vi "__Alicat SD_ManualSetFlows.vi"(1 "SET FLOW":dbl[](array[numeric])=[0.0, 0.0] format="%.2f", 6 "error in (no error)":errorcluster, 9 "COMMS":T1={"Alicats"="ASRL6::INSTR", "Alic"=FALSE, "eValve"="ASRL6::INSTR", "eval"=FALSE, "Eurotherm"="ASRL6::INSTR", "euro"=FALSE, "Cell GAS"="ASRL6::INSTR", "cgas"=FALSE, "Cell H2S"="ASRL6::INSTR", "ch2s"=FALSE}) -> (0 "error out":errorcluster, 3 "Cancelled?":bool)   [LabVIEW 2017]
doc: "Use this template to create a dialog box. This template polls the state of the buttons on the front panel and does not use events. Use the Dialog Using Events template (not available in Base package) to create a dialog box with event handling."
uses:
  __s_TablaAlicats.ctl
  REACTOR_COMUNICACIONES.ctl
  REACTOR_GLOBALES.vi
panel:
  in  "Canal4":bool
  in  "Canal3":bool
  out "ID":string[](array[string])
  out "CONECTADO":bool[](array[boolean])
  in  "Canal2":bool
  in  "Canal1":bool
  out "aDispositivos":T2=[["A", "NO", "aM0000013", "Air", "100", "ln/mn", "0.1", "0.11"], ["B", "NO", "aM0000014", "Air", "100", "ln/mn", "0.2", "0.22"], ["C", "NO", "aM0000015", "Air", "100", "ln/mn", "0.3", "0.33"], ["D", "NO", "aM0000016", "Air", "500", "ln/mn", "0.4", "0.44"]] caption="Alicats"
  out "RANGOS":dbl[](array[numeric]) format="%.1g"
  in  "Cancel":bool
  in  "OK":bool
  # "Nota: \nAl hacer CLICK en el botón aparecerá\nla ventana para establecer el nuevo setpoint"
  # "Flujos Alicats"
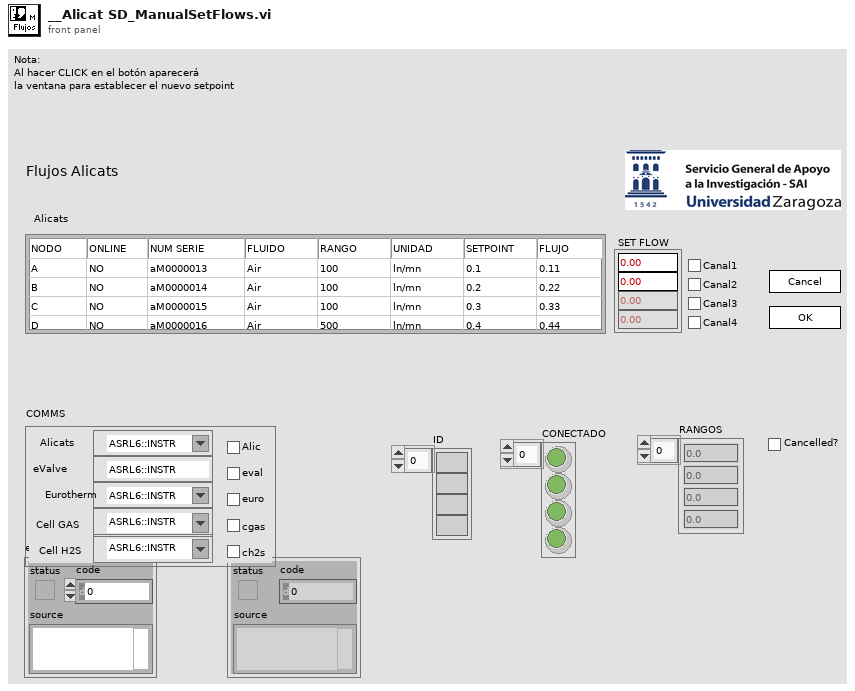
[diagram p1: front panel]
types:
  T1 = typedef "REACTOR_COMUNICACIONES.ctl" = cluster{"Alicats":refnum<visa-resource-name>, "Alic":bool, "eValve":refnum<visa-resource-name>, "eval":bool, "Eurotherm":refnum<visa-resource-name>, "euro":bool, "Cell GAS":refnum<visa-resource-name>, "cgas":bool, "Cell H2S":refnum<visa-resource-name>, "ch2s":bool}
  T2 = typedef "__s_TablaAlicats.ctl" = string[][]
  T3 = typedef "__s_SPali4.ctl" = cluster{"Ch1":dbl, "Ch2":dbl, "Ch3":dbl, "Ch4":dbl}
  T4 = cluster{"SETPOINT 2[0]":dbl, "SETPOINT 2[1]":dbl, "SETPOINT 2[2]":dbl, "SETPOINT 2[3]":dbl}
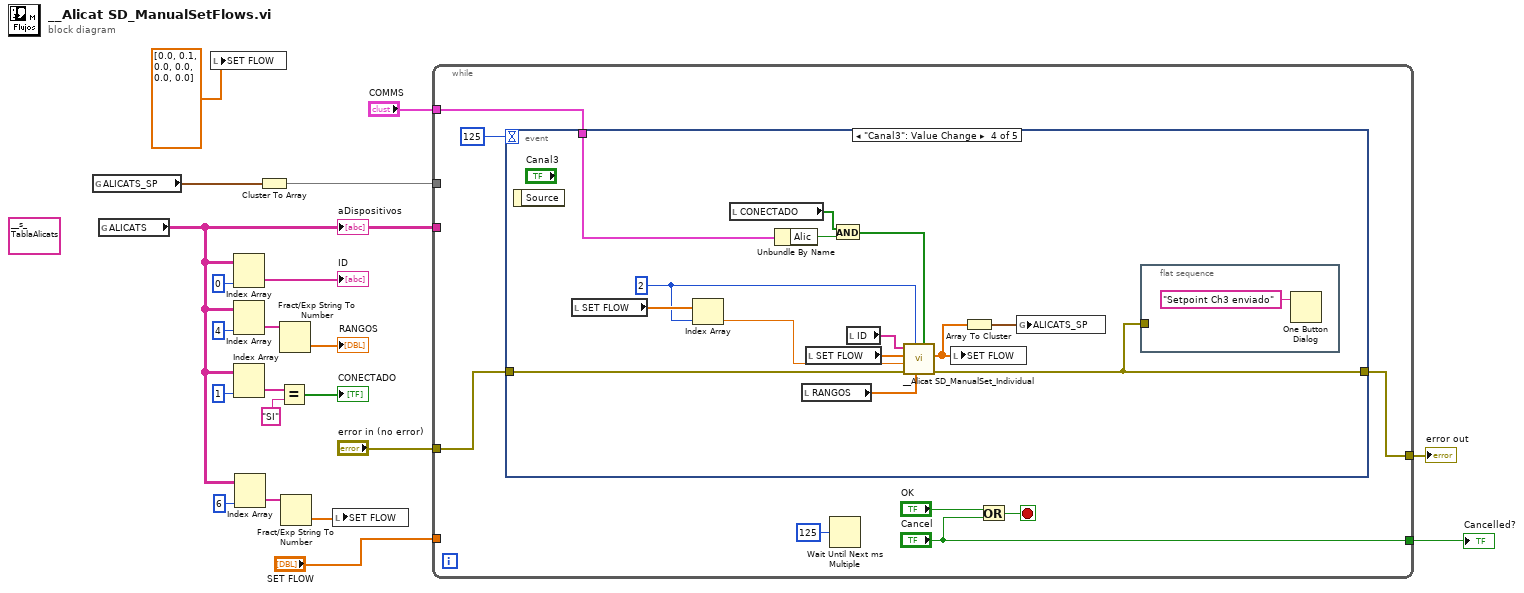
[diagram p0: block diagram]
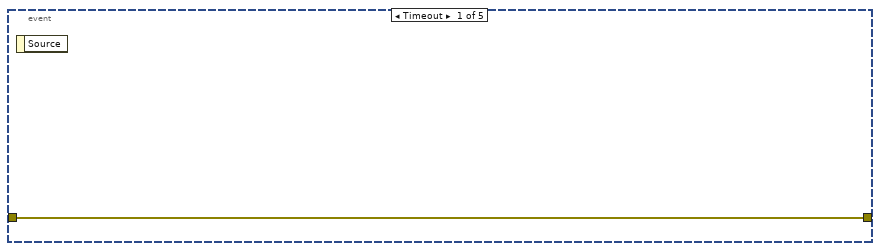
[diagram p2: hidden frame]
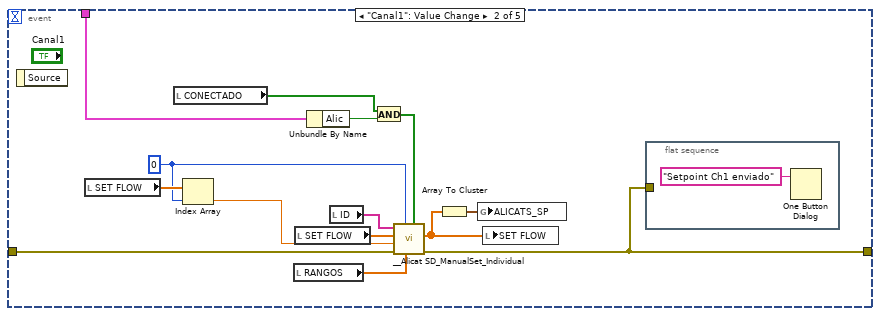
[diagram p3: hidden frame]
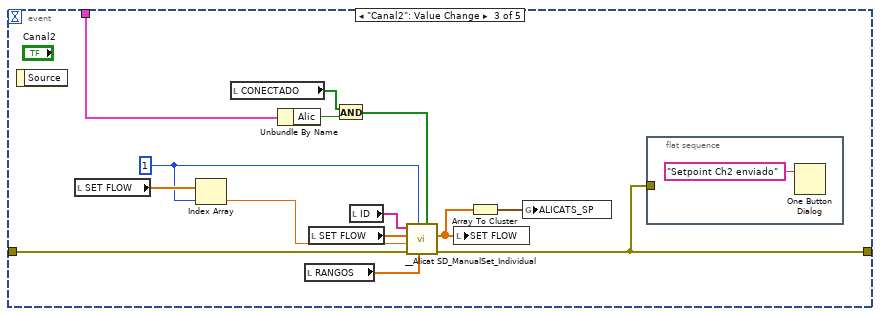
[diagram p4: hidden frame]
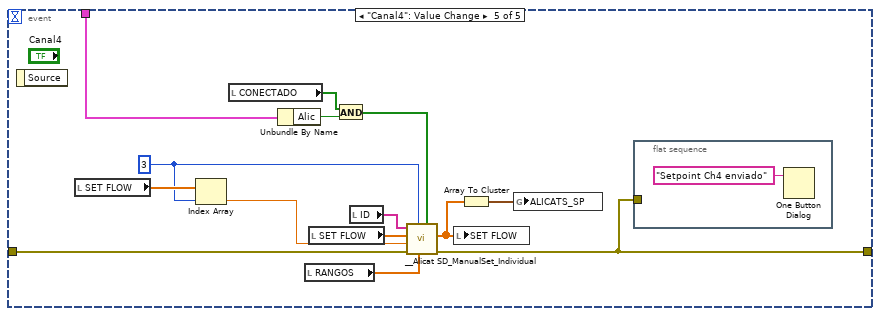
[diagram p5: hidden frame]
diagram:
  (unwired) T2 [["3", "NO", "aM0000013", "Air", "1", "ln/mn", "0.1", "0.11"], ["4", "NO", "aM0000014", "Air", "1", "ln/mn", "0.2", "0.22"], ["5", "NO", "aM0000015", "Air", "1", "ln/mn", "0.3", "0.33"], ["6", "NO", "aM0000016", "Air", "1", "ln/mn", "0.4", "0.44"]] ("Dispositivos 2")
  n1 = global read "REACTOR_GLOBALES.vi" "ALICATS_SP"() -> (w9:T3)
  n2 = global read "REACTOR_GLOBALES.vi" "ALICATS"() -> (w3:T2)
  "aDispositivos" <- w3
  n3 = local write "SET FLOW"(dbl[] [0.0, 0.1, 0.0, 0.0, 0.0, 0.0] ("SET FLOW")) -> ()
  n4 = Index Array(array=w3, index (col)=0 ("disabled index (col)")) -> (element=→"ID":string[])  [unwired: 1 in]
  n5 = Index Array(array=w3, index (col)=4 ("disabled index (col)")) -> (element=w19:string[])  [unwired: 1 in]
  n6 = Index Array(array=w3, index (col)=1 ("disabled index (col)")) -> (element=w12:string[])  [unwired: 1 in]
  n7 = Index Array(array=w3, index (col)=6 ("disabled index (col)")) -> (element=w5:string[])  [unwired: 1 in]
  n8 = Cluster To Array(cluster=w9) -> (array=w7:dbl[])
  n9 = Equal?(x=w12, y="SI") -> (x = y?=→"CONECTADO":bool[])
  n10 = Fract/Exp String To Number(string=w19) -> (number=→"RANGOS":dbl[])  [unwired: 3 in, 1 out]
  n11 = Fract/Exp String To Number(string=w5) -> (number=w1:dbl[])  [unwired: 3 in, 1 out]
  n12 = local write "SET FLOW"(w1) -> ()
  n13 = while {
    tunnel: ["Cancel"] -> w21
    tunnel: "error in (no error)" -> [w24]
    tunnel: [w23] -> w16
    tunnel: w3 -> [_]
    tunnel: "COMMS" -> [w22]
    tunnel: w7 -> [_]
    tunnel: "SET FLOW" -> [_]
    stop <- w28 stop-if-true
    n14 = event shown="[3] \"Canal3\": Value Change" {
      selector: _ -> [_ _ _ _ _]
      dyn-events: _ -> [_ _ _ _ _]
      timeout: 125 -> [_ _ _ _ _]
      tunnel: w24 -> [w30 w32 w47 w63 w78]
      tunnel: [w30 w31 w46 w61 w76] -> w23
      tunnel: w22 -> [_ w34 w49 w64 w79]
      event Timeout {
        n15 = event-data() -> ()  [unwired: 1 in, 1 out]
      }
      event "Canal1": Value Change {
        w40 = 0 ("Address (0.7)")
        n16 = event-data() -> ()  [unwired: 1 in, 1 out]
        n17 = local read "SET FLOW"() -> (w41:dbl[])
        n18 = local read "CONECTADO"() -> (w38:bool[])
        n19 = Index Array(array=w41, index=w40) -> (element=w33:dbl)
        n20 = local read "RANGOS"() -> (w44:dbl[])
        n21 = local read "SET FLOW"() -> (w43:dbl[])
        n22 = Unbundle By Name(w34) -> ("Alic"=w39:bool)
        n23 = local read "ID"() -> (w42:string[])
        n24 = And(x=w38, y=w39) -> (x .and. y?=w37:bool[])
        n25 = call "__Alicat SD_ManualSet_Individual.vi"("USADO"=w37, "RANGOS"=w44, "Address (0.7)"=w40, "error in"=w32, 9:"SETPOINT"=w33, 10:"SETPOINT"=w43, "ID"=w42) -> ("error out"=w31:errorcluster, "SETPOINT 2"=w36:dbl[])  [unwired: 3 in]
        n26 = Array To Cluster(array=w36) -> (cluster=w35:T4)
        n27 = global write "REACTOR_GLOBALES.vi" "ALICATS_SP"(w35) -> ()
        n28 = local write "SET FLOW"(w36) -> ()
        n29 = flat-sequence {
          tunnel: w31 -> [_]
          frame #0 {
            n30 = One Button Dialog(message="Setpoint Ch1 enviado") -> ()  [unwired: 1 in, 1 out]
          }
        }
      }
      event "Canal2": Value Change {
        w55 = 1 ("Address (0.7)")
        n31 = event-data() -> ()  [unwired: 1 in, 1 out]
        n32 = local read "SET FLOW"() -> (w56:dbl[])
        n33 = Index Array(array=w56, index=w55) -> (element=w48:dbl)
        n34 = local read "CONECTADO"() -> (w53:bool[])
        n35 = Unbundle By Name(w49) -> ("Alic"=w54:bool)
        n36 = local read "RANGOS"() -> (w59:dbl[])
        n37 = local read "SET FLOW"() -> (w58:dbl[])
        n38 = And(x=w53, y=w54) -> (x .and. y?=w52:bool[])
        n39 = local read "ID"() -> (w57:string[])
        n40 = call "__Alicat SD_ManualSet_Individual.vi"("USADO"=w52, "RANGOS"=w59, "Address (0.7)"=w55, "error in"=w47, 9:"SETPOINT"=w48, 10:"SETPOINT"=w58, "ID"=w57) -> ("error out"=w46:errorcluster, "SETPOINT 2"=w50:dbl[])  [unwired: 3 in]
        n41 = local write "SET FLOW"(w50) -> ()
        n42 = Array To Cluster(array=w50) -> (cluster=w51:T4)
        n43 = global write "REACTOR_GLOBALES.vi" "ALICATS_SP"(w51) -> ()
        n44 = flat-sequence {
          tunnel: w46 -> [_]
          frame #0 {
            n45 = One Button Dialog(message="Setpoint Ch2 enviado") -> ()  [unwired: 1 in, 1 out]
          }
        }
      }
      event "Canal3": Value Change {
        w70 = 2 ("Address (0.7)")
        n46 = event-data() -> ()  [unwired: 1 in, 1 out]
        n47 = local read "SET FLOW"() -> (w71:dbl[])
        n48 = Index Array(array=w71, index=w70) -> (element=w62:dbl)
        n49 = local read "CONECTADO"() -> (w68:bool[])
        n50 = Unbundle By Name(w64) -> ("Alic"=w69:bool)
        n51 = local read "RANGOS"() -> (w74:dbl[])
        n52 = local read "SET FLOW"() -> (w73:dbl[])
        n53 = And(x=w68, y=w69) -> (x .and. y?=w67:bool[])
        n54 = local read "ID"() -> (w72:string[])
        n55 = call "__Alicat SD_ManualSet_Individual.vi"("USADO"=w67, "RANGOS"=w74, "Address (0.7)"=w70, "error in"=w63, 9:"SETPOINT"=w62, 10:"SETPOINT"=w73, "ID"=w72) -> ("error out"=w61:errorcluster, "SETPOINT 2"=w65:dbl[])  [unwired: 3 in]
        n56 = local write "SET FLOW"(w65) -> ()
        n57 = Array To Cluster(array=w65) -> (cluster=w66:T4)
        n58 = global write "REACTOR_GLOBALES.vi" "ALICATS_SP"(w66) -> ()
        n59 = flat-sequence {
          tunnel: w61 -> [_]
          frame #0 {
            n60 = One Button Dialog(message="Setpoint Ch3 enviado") -> ()  [unwired: 1 in, 1 out]
          }
        }
      }
      event "Canal4": Value Change {
        w85 = 3 ("Address (0.7)")
        n61 = event-data() -> ()  [unwired: 1 in, 1 out]
        n62 = local read "SET FLOW"() -> (w86:dbl[])
        n63 = Index Array(array=w86, index=w85) -> (element=w77:dbl)
        n64 = local read "CONECTADO"() -> (w83:bool[])
        n65 = Unbundle By Name(w79) -> ("Alic"=w84:bool)
        n66 = local read "RANGOS"() -> (w89:dbl[])
        n67 = local read "SET FLOW"() -> (w88:dbl[])
        n68 = And(x=w83, y=w84) -> (x .and. y?=w82:bool[])
        n69 = local read "ID"() -> (w87:string[])
        n70 = call "__Alicat SD_ManualSet_Individual.vi"("USADO"=w82, "RANGOS"=w89, "Address (0.7)"=w85, "error in"=w78, 9:"SETPOINT"=w77, 10:"SETPOINT"=w88, "ID"=w87) -> ("error out"=w76:errorcluster, "SETPOINT 2"=w80:dbl[])  [unwired: 3 in]
        n71 = local write "SET FLOW"(w80) -> ()
        n72 = Array To Cluster(array=w80) -> (cluster=w81:T4)
        n73 = global write "REACTOR_GLOBALES.vi" "ALICATS_SP"(w81) -> ()
        n74 = flat-sequence {
          tunnel: w76 -> [_]
          frame #0 {
            n75 = One Button Dialog(message="Setpoint Ch4 enviado") -> ()  [unwired: 1 in, 1 out]
          }
        }
      }
    }
    n76 = Wait Until Next ms Multiple(millisecond multiple=u32 125) -> ()  [unwired: 1 out]
    n77 = Or(x="OK", y="Cancel") -> (x .or. y?=w28:bool)
  }
  "Cancelled?" <- w21
  "error out" <- w16
